vi "POI Averaging.vi"(9 "Data in":T1) -> (1 "Data out":T1, 3 "Averaged":bool)   [LabVIEW 2020]
uses:
  xcontrol/Interface VIs/Interface typedefs/Interface-Data array.ctl
  xcontrol/Interface VIs/Interface typedefs/Interface-Data format definition.ctl
  xcontrol/Typedefs/Xctl-XY data type definition.ctl
  xcontrol/Typedefs/Xctrl-ROI type enum.ctl
  <vilib>/Analysis/baseanly.llb/Mean (DBL).vi
  <vilib>/Analysis/NI_AALBase.lvlib
  xcontrol/XGrapher.xctl
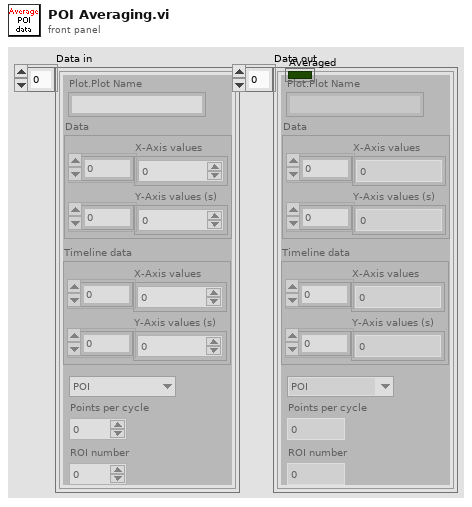
[diagram p1: front panel]
types:
  T1 = typedef "Interface-Data array.ctl" = T2[]
  T2 = typedef "Interface-Data format definition.ctl" = cluster{"Plot.Plot Name":string, "Data":T3, "Timeline data":T3, "Type":T4, "Points per cycle":u16, "ROI number":u16}
  T3 = typedef "XGrapher.xctl/Xctl-XY data type definition.ctl" = cluster{"X-Axis values":sgl[], "Y-Axis values (s)":sgl[]}
  T4 = typedef "Xctrl-ROI type enum.ctl" = enum16{"POI", "Mini-scan", "Group"}
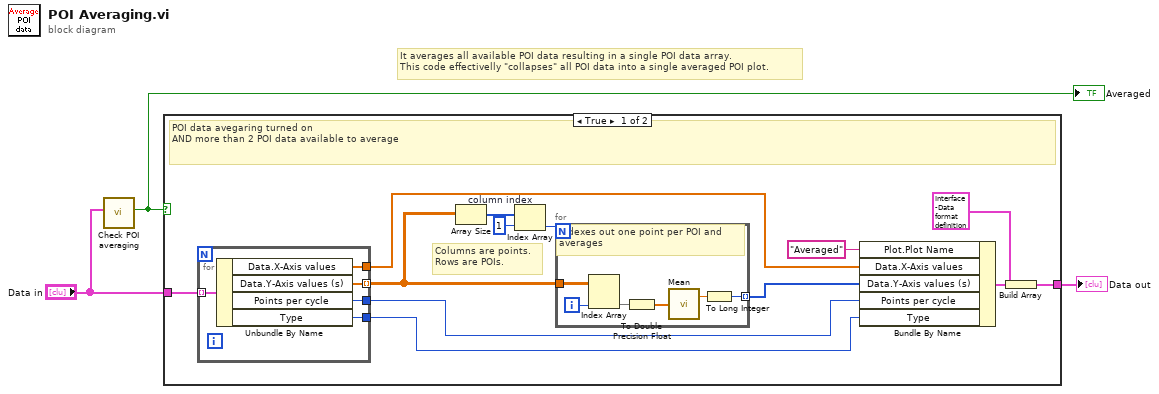
[diagram p0: block diagram]
diagram:
  # "It averages all available POI data resulting in a single POI data array.\nThis code effectivelly \"collapses\" all POI data into a single averaged POI plot."
  n1 = call "Check POI averaging.vi"("Data in"="Data in") -> ("Average"=w1:bool)  [unwired: 10 in]
  "Averaged" <- w1
  n2 = case shown="True" w1 {
    tunnel: "Data in" -> [w16 w28]
    tunnel: [w15 w28] -> w3
    frame True {
      w13 = 1  # column index
      # "Columns are points.\nRows are POIs."
      # "POI data avegaring turned on\nAND more than 2 POI data available to average"
      n3 = for {
        tunnel: w16 -> [w21] mode=indexing
        tunnel: [w20] -> w11 mode=indexing
        tunnel: [w19] -> w9
        tunnel: [w18] -> w5
        tunnel: [w17] -> w6
        n4 = Unbundle By Name(w21) -> ("Data.X-Axis values"=w18:sgl[], "Data.Y-Axis values (s)"=w20:sgl[], "Points per cycle"=w19:u16, "Type"=w17:T4)
      }
      n5 = Array Size(array=w11) -> (size(s)=w14:i32[])
      n6 = Index Array(array=w14, index=w13) -> (element=w12:i32)
      n7 = for {
        N: w12 -> [_]
        tunnel: w11 -> [w26]
        tunnel: [w22] -> w4 mode=indexing
        i -> [w27]
        # "Indexes out one point per POI and averages"
        n8 = Index Array(array=w26, index (col)=w27) -> (element=w25:sgl[])  [unwired: 1 in]
        n9 = To Double Precision Float(number=w25) -> (double precision float=w23:dbl[])
        n10 = call-poly <vilib>:"Mean.vi"("X"=w23) -> ("mean"=w24:dbl)  [unwired: 1 out]
        n11 = To Long Integer(number=w24) -> (32bit integer=w22:i32)
      }
      n12 = Bundle By Name(cluster=T2 {"Plot.Plot Name"="", "Data"={"X-Axis values"=[], "Y-Axis values (s)"=[]}, "Timeline data"={"X-Axis values"=[], "Y-Axis values (s)"=[]}, "Type"=enum."POI", "Points per cycle"=0, "ROI number"=0}, "Plot.Plot Name"="Averaged", "Data.X-Axis values"=w5, "Data.Y-Axis values (s)"=w4, "Points per cycle"=w9, "Type"=w6) -> (w10:T2)
      n13 = Build Array(w10) -> (w15:T2[])
    }
    frame False {
      # "POI data avegaring turned off\nOR less than 2 POI datasets available"
    }
  }
  "Data out" <- w3
